vi "GenerateCode.vi"(1 "Terms":T1[](array[typedef]), 3 "Diagram":refnum<vi>, 5 "XRef":refnum<vi>, 6 "State In":T4={"Enum Type"=variant(dbl 0.0), "Types Type"=variant, "Enum Names"=[], "Type Names"=[], "Typedef Name"="", "Typedef Path"=path ""}) -> (0 "Generated Code?":bool, 2 "State Out":T4={"Enum Type"=variant(dbl 0.0), "Types Type"=variant, "Enum Names"=[], "Type Names"=[], "Typedef Name"="", "Typedef Path"=path ""}, 4 "Reply":string[](array[string]))   [LabVIEW 2015, in "Define-Tagged-Union.xnode"]
doc: "This ability VI is called when it is time to define the execution behavior of your XNode via LabVIEW's scripting API. This VI is only called when you have previously informed LabVIEW that you need to script through a GenerateCode reply. Diagram is a reference to a diagram of a temporary VI. This diagram contains exactly one front panel terminal for each terminal of your XNode. Terms is an array of pairs of Term IDs and terminal references. LabVIEW will copy code scripted into this diagram into your XNode and connect everything to the correct terminals. The front panel terminals that are on this diagram are special in that they can only be on the top level diagram.\n \n Generate Code? is used to tell LabVIEW whether or not you want to copy the scripted diagram over. If there is an error and you wish not to commit the changes, then the old XNode behavior will be left unchanged. If you set Generate Code? to false, then this VI will be called again next time type propagation is run. Otherwise, it will not be called until you indicate that it should be through the reply on another ability VI.\n \n Because the diagram you are scripting into is separate from the VI containing the XNode instance, type propagation and the data manager will run on the temporary VI after each scripting call.\n \n You should not use the Copy scripting method to move code into the temporary VI. This will adversely affect the user's clipboard. You should use the Move scripting method instead.\n\nDefault behavior: None.\n\nThis ability does not provide UI and OS messages are not handled.\n\nSee also: ModifyCode"
uses:
  Define-Tagged-Union.xnode
  State.ctl
  <vilib>/XNodeSupport/XNodeTermIDPair.ctl
  <vilib>/XNodeSupport/XNodeTermRef.ctl
  <vilib>/XNodeSupport/XNodeString.ctl
  <vilib>/Erdos Miller/LV-Scripting/LV-Scripting.lvlib
  <vilib>/Utility/Data Type/NI_Data Type.lvlib
  <vilib>/XNodeSupport/NI_XNodeSupport.lvlib
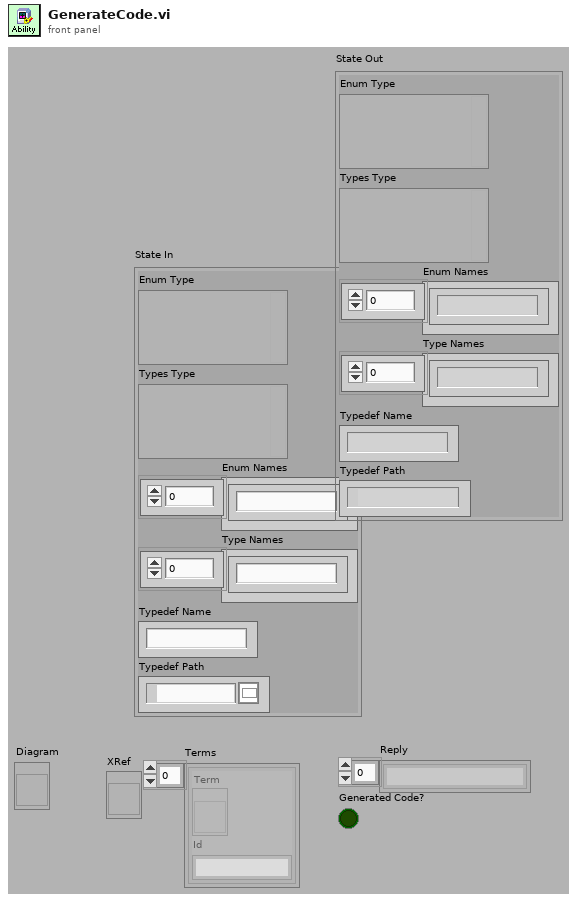
[diagram p1: front panel]
types:
  T1 = typedef "NI_XNodeSupport.lvlib/XNodeTermIDPair.ctl" = cluster{"Term":T2, "Id":T3}
  T2 = typedef "NI_XNodeSupport.lvlib/XNodeTermRef.ctl" = refnum<vi>
  T3 = typedef "NI_XNodeSupport.lvlib/XNodeString.ctl" = string
  T4 = typedef "Define-Tagged-Union.xnode/State.ctl" = cluster{"Enum Type":variant, "Types Type":variant, "Enum Names":string[], "Type Names":string[], "Typedef Name":string, "Typedef Path":path}
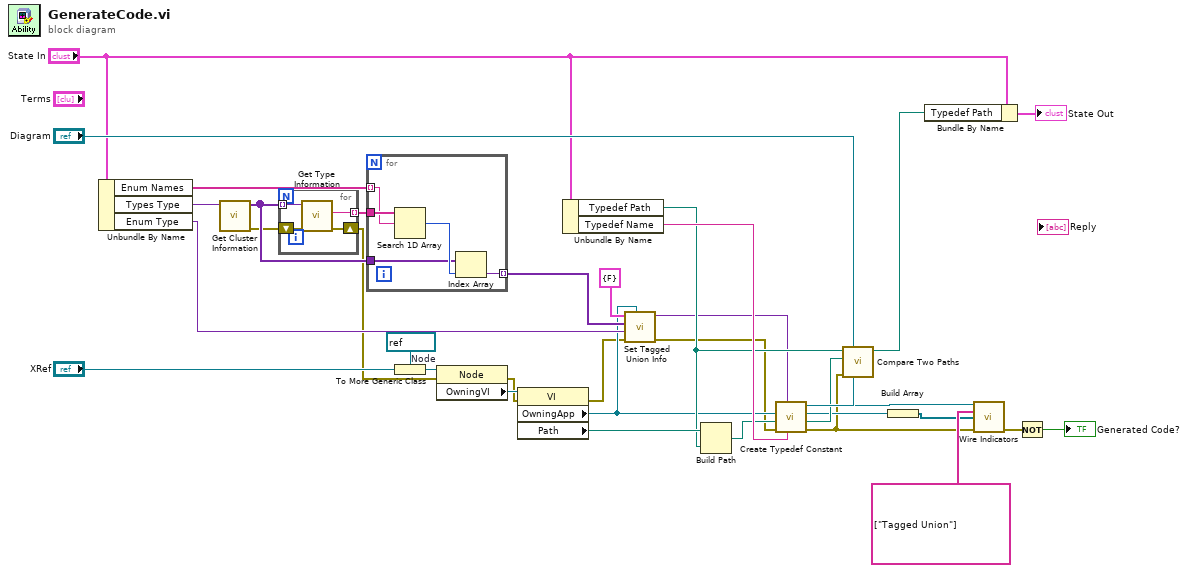
[diagram p0: block diagram]
diagram:
  w34 = refnum<vi> refnum  # Node
  n1 = Unbundle By Name("State In") -> ("Enum Names"=w19:string[], "Types Type"=w20:variant, "Enum Type"=w13:variant)
  n2 = call <vilib>:"Get Cluster Information.vi"("Variant"=w20) -> ("error out"=w16:errorcluster, "Cluster Elements"=w18:variant[])  [unwired: 9 in]
  n3 = for {
    tunnel: w18 -> [w38] mode=indexing
    tunnel: [w37] -> w17 mode=indexing
    shift-right: [w35] -> w4
    shift-left: w16 -> [w36]
    n4 = call <vilib>:"Get Type Information.vi"("error in (no error)"=w36, "Variant"=w38) -> ("error out"=w35:errorcluster, "Name"=w37:string)  [unwired: 5 in, 3 out]
  }
  n5 = for {
    tunnel: w19 -> [w42] mode=indexing
    tunnel: w18 -> [w40]
    tunnel: w17 -> [w43]
    tunnel: [w39] -> w14 mode=indexing
    n6 = Search 1D Array(1D array=w43, element=w42) -> (index of element=w41:i32)  [unwired: 1 in]
    n7 = Index Array(array=w40, index=w41) -> (element=w39:variant)
  }
  n8 = To More Generic Class(target class=w34, reference="XRef") -> (generic class reference=w33:refnum<vi>)
  n9 = property class="Node"(reference=w33, error in=w4) -> (error out=w11:errorcluster, "OwningVI"=w32:refnum<vi>)  [unwired: 1 out]
  n10 = property class="VI"(reference=w32, error in=w11) -> (error out=w2:errorcluster, "OwningApp"=w3:refnum<vi>, "Path"=w26:path)  [unwired: 1 out]
  n11 = Unbundle By Name("State In") -> ("Typedef Path"=w24:path, "Typedef Name"=w29:string)
  n12 = call <vilib>:"Set Tagged Union Info.vi"("application reference (local)"=w3, "error in (no error)"=w2, "Enum Type"=w13, "Element Types"=w14, "Variant in"=cluster{bool} {FALSE}) -> ("error out"=w1:errorcluster, "Variant out"=w12:variant)  [unwired: 5 in]
  n13 = Build Path(base path=w26, name or relative path=w24) -> (appended path=w25:path)
  n14 = call <vilib>:"Create Typedef Constant.vi"("Typedef Name"=w29, "Type"=w12, "error in (no error)"=w1, "Typedef Path"=w25, "Application"=w3, "Diagram in"="Diagram") -> ("error out"=w7:errorcluster, "New Typedef Path"=w23:path, "Constant"=w9:refnum<vi>, "Diagram out"=w10:refnum<vi>)  [unwired: 2 in]
  n15 = call <vilib>:"Compare Two Paths.vi"("error in (no error)"=w7, "Path 2"=w23, "Path 1"=w24) -> ("Relative Path from 1 to 2"=w22:path)  [unwired: 5 in, 3 out]
  n16 = Build Array(w9) -> (w8:refnum<vi>[])
  n17 = Bundle By Name(cluster="State In", "Typedef Path"=w22) -> (→"State Out":T4)
  n18 = call <vilib>:"Wire Indicators.vi"("Diagram in"=w10, "Indicator Names"=string[] ["Tagged Union"], "Outputs"=w8, "error in (no error)"=w7) -> ("error out"=w6:errorcluster)  [unwired: 10 in, 1 out]
  n19 = Not(x=w6) -> (.not. x?=→"Generated Code?":bool)
